vi "AverageXYZ (SubVI) 1.vi"(8 "array":dbl[][][](array[numeric])) -> (0 "Bottom SD":dbl[][](array[numeric]), 1 "Bottom averages":dbl[][](array[numeric]), 2 "Top SD":dbl[][](array[numeric]), 3 "Top averages":dbl[][](array[numeric]))   [LabVIEW 2016]
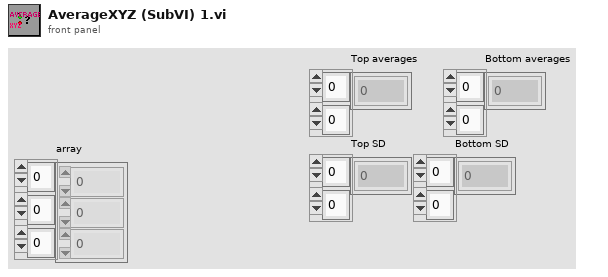
[diagram p1: front panel]
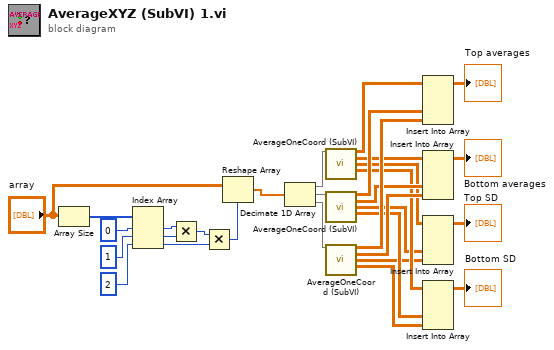
[diagram p0: block diagram]
diagram:
  n1 = Array Size(array="array") -> (size(s)=w27:i32[])
  n2 = Index Array(array=w27, index #1=0 ("index"), index #2=1 ("index"), index #3=2 ("index")) -> (element #1=w23:i32, element #2=w22:i32, element #3=w20:i32)
  n3 = Multiply(x=w23, y=w22) -> (x*y=w21:i32)
  n4 = Multiply(x=w21, y=w20) -> (x*y=w18:i32)
  n5 = Reshape Array("array", w18) -> (w17:dbl[])
  n6 = Decimate 1D Array(w17) -> (w30:dbl[], w29:dbl[], w28:dbl[])
  n7 = call "AverageOneCoord (SubVI).vi"("Array"=w30) -> ("Top averages"=w16:dbl[][], "Bottom averages"=w13:dbl[][], "Top SD"=w10:dbl[][], "Bottom SD"=w9:dbl[][])  [unwired: 11 in]
  n8 = call "AverageOneCoord (SubVI).vi"("Array"=w29) -> ("Top averages"=w15:dbl[][], "Bottom averages"=w12:dbl[][], "Top SD"=w8:dbl[][], "Bottom SD"=w7:dbl[][])  [unwired: 11 in]
  n9 = call "AverageOneCoord (SubVI).vi"("Array"=w28) -> ("Top averages"=w14:dbl[][], "Bottom averages"=w11:dbl[][], "Top SD"=w6:dbl[][], "Bottom SD"=w5:dbl[][])  [unwired: 11 in]
  n10 = Insert Into Array(array=w16, new element #1=w15, new element #2=w14) -> (→"Top averages":dbl[][])  [unwired: 2 in]
  n11 = Insert Into Array(array=w13, new element #1=w12, new element #2=w11) -> (→"Bottom averages":dbl[][])  [unwired: 2 in]
  n12 = Insert Into Array(array=w10, new element #1=w8, new element #2=w6) -> (→"Top SD":dbl[][])  [unwired: 2 in]
  n13 = Insert Into Array(array=w9, new element #1=w7, new element #2=w5) -> (→"Bottom SD":dbl[][])  [unwired: 2 in]
